vi "Confirm Device UI.vi"(11 "Device":refnum<class "Device.lvclass">) -> (3 "Confirmed":bool)   [LabVIEW 2020, in "PicoG-App.lvlib" / "App.lvclass"]
uses:
  App.lvclass
  Device/Device.lvclass
panel:
  in  "Cancel Button":bool
  in  "OK Button":bool
  out "Version":string
  out "Alias":string
  out "Id / Serial":string
  out "Board":string
  out "Platform":string
  # "Confirm device selection to continue adding the device to the registry.\n\nIf desired, the alias can be changed once the device is added."
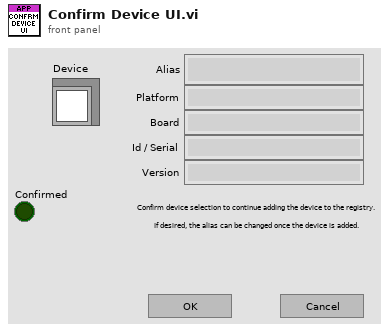
[diagram p1: front panel]
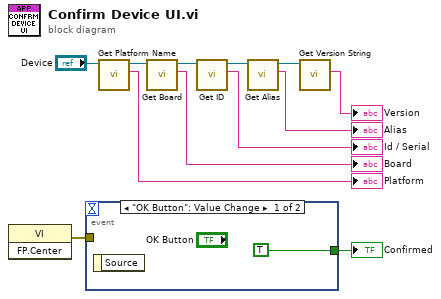
[diagram p0: block diagram]
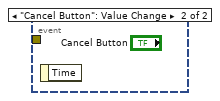
[diagram p2: hidden frame]
diagram:
  n1 = invoke class="VI" method="FP.Center"() -> (error out=w1:errorcluster)  [unwired: 3 in, 2 out]
  n2 = event shown="[0] \"OK Button\": Value Change" {
    selector: _ -> [_ _]
    dyn-events: _ -> [_ _]
    timeout: _ -> [_ _]
    tunnel: [TRUE _] -> w2
    tunnel: w1 -> [_ _]
    event "OK Button": Value Change {
      n3 = event-data() -> ()  [unwired: 1 in, 1 out]
    }
    event "Cancel Button": Value Change {
      n4 = event-data() -> ()  [unwired: 1 in, 1 out]
    }
  }
  "Confirmed" <- w2
  n5 = call "Get Platform Name.vi"("Device in"="Device") -> ("Platform"=→"Platform":string, "Device out"=w11:refnum<class "Device.lvclass">)  [unwired: 8 in, 1 out]
  n6 = call "Get Board.vi"("Device in"=w11) -> ("Board"=→"Board":string, "Device out"=w10:refnum<class "Device.lvclass">)  [unwired: 8 in, 1 out]
  n7 = call "Get ID.vi"("Device in"=w10) -> ("Id"=→"Id / Serial":string, "Device out"=w9:refnum<class "Device.lvclass">)  [unwired: 8 in, 1 out]
  n8 = call "Get Alias.vi"("Device in"=w9) -> ("Alias"=→"Alias":string, "Device out"=w8:refnum<class "Device.lvclass">)  [unwired: 8 in, 1 out]
  n9 = call "Get Version String.vi"("Device in"=w8) -> ("Version"=→"Version":string)  [unwired: 8 in, 2 out]
